vi "setup.vi"() -> (2 "Data":T1={"Report.lvclass"=refnum, "test"="", "last State"=enum."Initialize", "test ID"=0, "parameter"=[], "EMTestCWS500N.lvclass"=refnum, "CEG4500.lvclass"=refnum, "Tektronix RSA5106A.lvclass"=refnum, "erfolgreich"=FALSE, "log"="", "Kommentar"="", "Device Enum"=enum."emTestCWS500N", "Test Enum"=enum."HF-Felder", "debug"=FALSE}, 3 "reference":refnum<vi>)   [LabVIEW 2013]
uses:
  Main/controls/Data.ctl
  classes/Datastructure/Report/Report.lvclass
  classes/Devices/emTestCWS500N/EMTestCWS500N.lvclass
  classes/Devices/CEG4500/CEG4500.lvclass
  classes/Devices/Tektronix RSA5106A/Tektronix RSA5106A.lvclass
  Main/controls/State.ctl
  classes/Devices/DeviceInterface/Devices.ctl
  classes/Tests/TestInterface/Tests.ctl
  classes/Datastructure/Norm/Norm.lvclass
  classes/Datastructure/Test/Test.lvclass
  classes/Datastructure/Image/img.lvclass
  classes/Datastructure/Setup/Setup.lvclass
  classes/Datastructure/Device/Device.lvclass
panel:
  in  "gelesen von Datenstruktur":string(tree)
  out "Fehler (Ausgang)":errorcluster
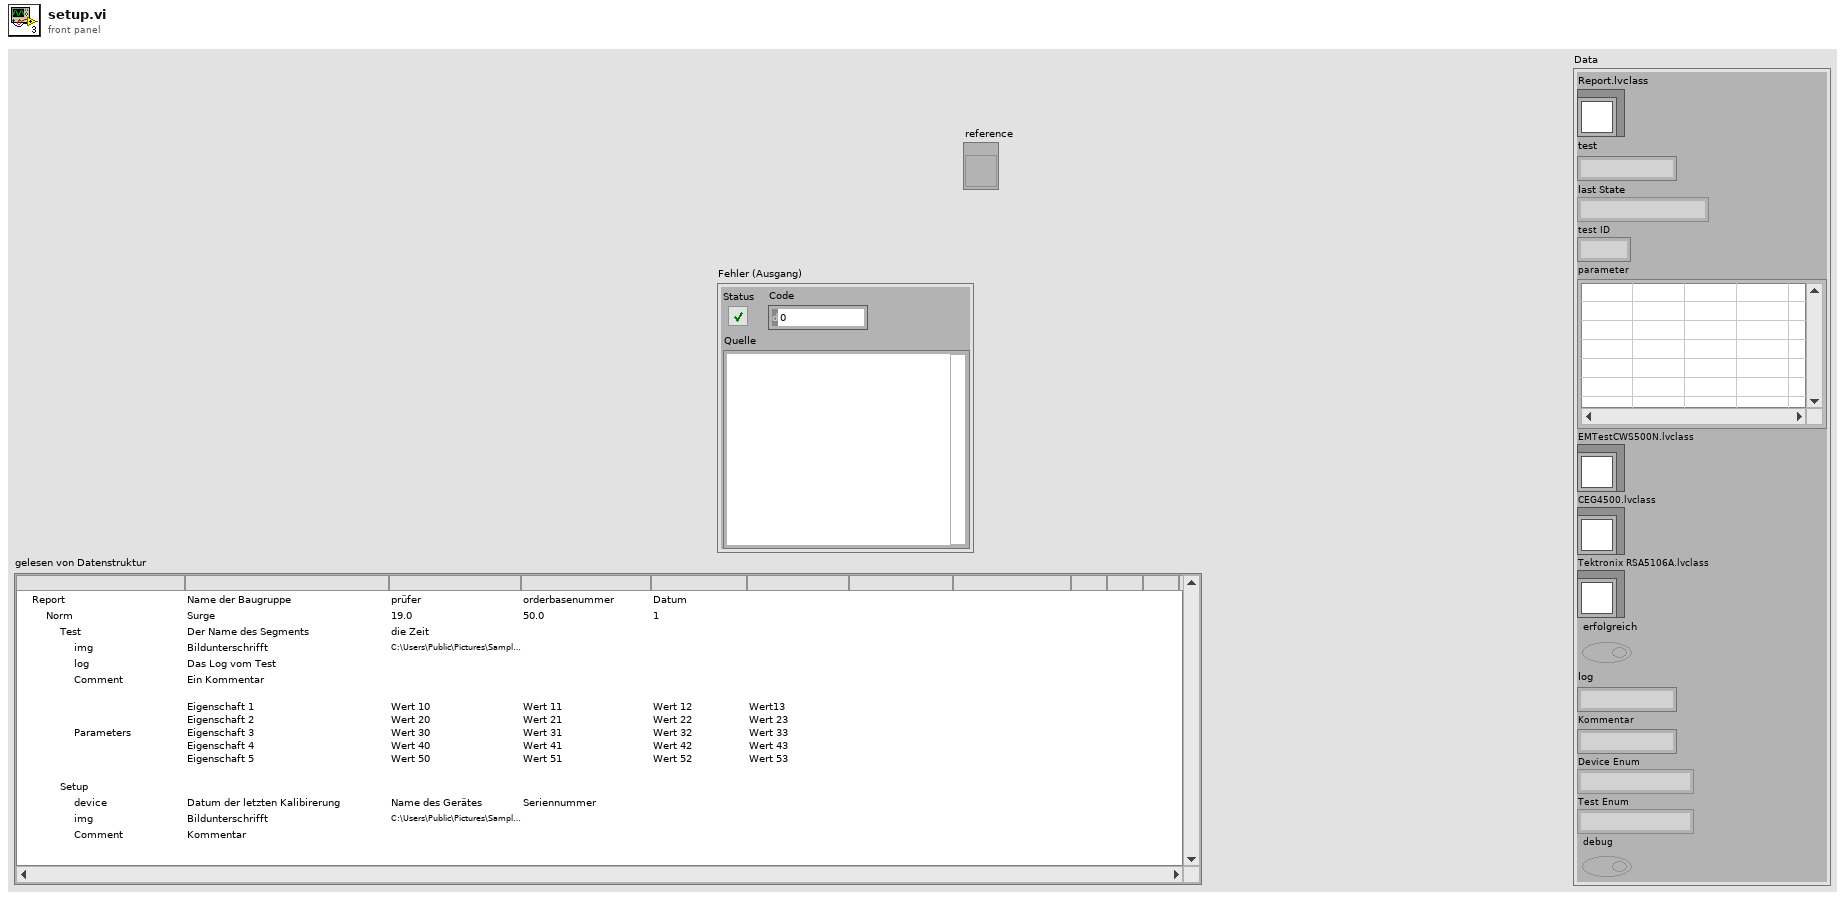
[diagram p1: front panel]
types:
  T1 = typedef "Data.ctl" = cluster{"Report.lvclass":refnum<class "Report.lvclass">, "test":string, "last State":T2, "test ID":i32, "parameter":string[][], "EMTestCWS500N.lvclass":refnum<class "EMTestCWS500N.lvclass">, "CEG4500.lvclass":refnum<class "CEG4500.lvclass">, "Tektronix RSA5106A.lvclass":refnum<class "Tektronix RSA5106A.lvclass">, "erfolgreich":bool, "log":string, "Kommentar":string, "Device Enum":T3, "Test Enum":T4, "debug":bool}
  T2 = typedef "State.ctl" = enum16{"create Pdf", "load Report", "save Report", "do Test", "CDN Kalibrierung", "enter Report Parameters", "new Test", "Protokoll", "read Tree", "update Tree", "Fehler", "Initialize", "Wait for Event", "Exit"}
  T3 = typedef "Devices.ctl" = enum16{"unbekannt", "Tektronix RSA5106A", "emTestCWS500N", "CEG-4500"}
  T4 = typedef "Tests.ctl" = enum16{"unbekannt", "Störaussendung", "Burst", "ESD", "Surge", "Spannungseinbruch", "HF-Felder"}
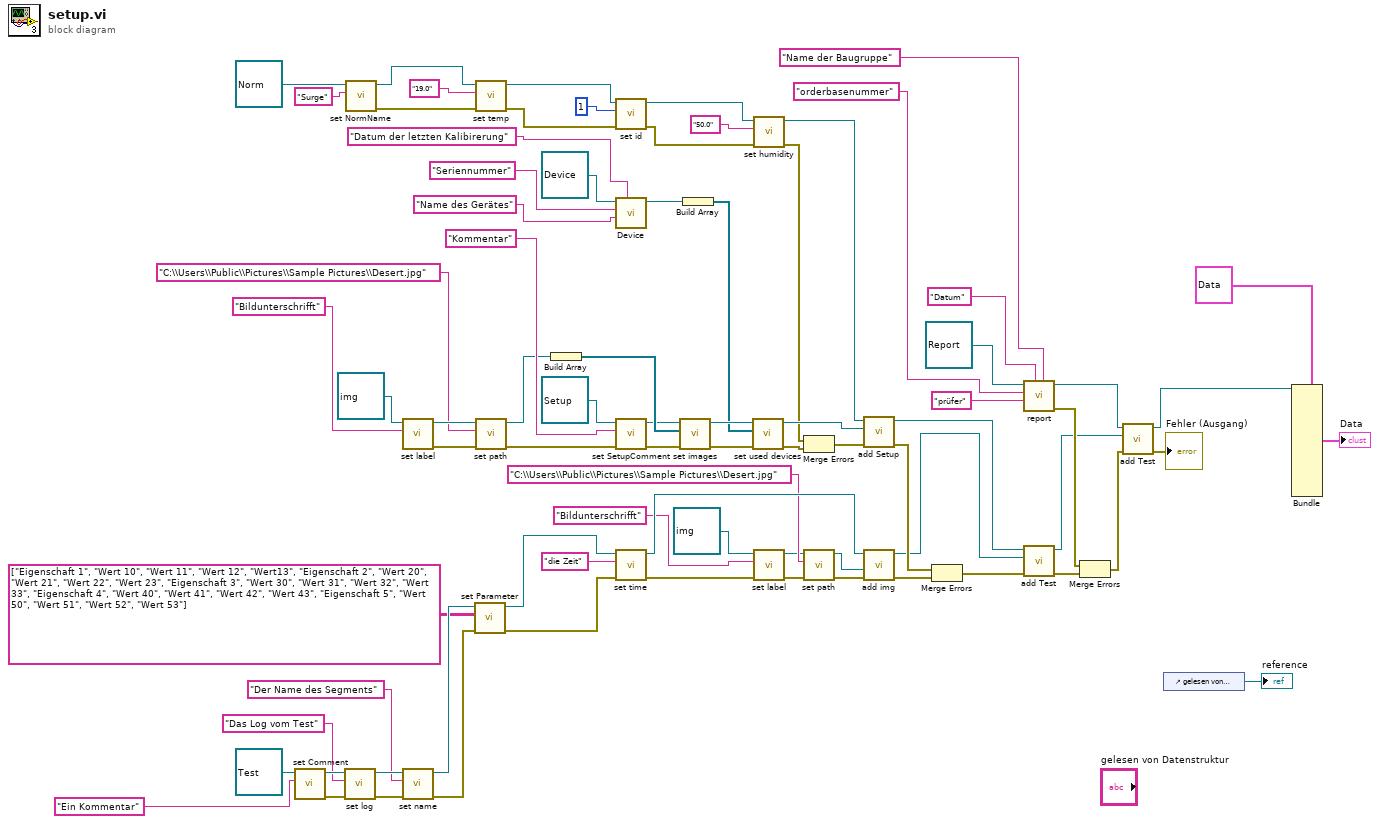
[diagram p0: block diagram]
diagram:
  n1 = call-dynamic "set Comment.vi"("Comment"="Ein Kommentar", "Segment (Eingang)"=refnum<class "Test.lvclass"> refnum ("Segment.lvclass")) -> ("error out"=w57:errorcluster, "Segment (Ausgang)"=w64:refnum<class "Test.lvclass">)  [unwired: 8 in]
  n2 = call-dynamic "set log.vi"("error in (no error)"=w57, "log"="Das Log vom Test", "Segment (Eingang)"=w64) -> ("error out"=w58:errorcluster, "Segment (Ausgang)"=w63:refnum<class "Test.lvclass">)  [unwired: 7 in]
  n3 = call-dynamic "set NormName.vi"("name"="Surge", "Test (Eingang)"=refnum<class "Norm.lvclass"> refnum ("Test.lvclass")) -> ("error out"=w8:errorcluster, "Test (Ausgang)"=w9:refnum<class "Norm.lvclass">)  [unwired: 8 in]
  n4 = call-dynamic "set label.vi"("label"="Bildunterschrifft", "img (Eingang)"=refnum<class "img.lvclass"> refnum ("img.lvclass")) -> ("error out"=w42:errorcluster, "img (Ausgang)"=w41:refnum<class "img.lvclass">)  [unwired: 8 in]
  n5 = call-dynamic "set name.vi"("error in (no error)"=w58, "name"="Der Name des Segments", "Segment (Eingang)"=w63) -> ("error out"=w59:errorcluster, "Segment (Ausgang)"=w62:refnum<class "Test.lvclass">)  [unwired: 7 in]
  n6 = call-dynamic "set Parameter.vi"("error in (no error)"=w59, "Parameter"=string[][] [["Eigenschaft 1", "Wert 10", "Wert 11", "Wert 12", "Wert13"], ["Eigenschaft 2", "Wert 20", "Wert 21", "Wert 22", "Wert 23"], ["Eigenschaft 3", "Wert 30", "Wert 31", "Wert 32", "Wert 33"], ["Eigenschaft 4", "Wert 40", "Wert 41", "Wert 42", "Wert 43"], ["Eigenschaft 5", "Wert 50", "Wert 51", "Wert 52", "Wert 53"]], "Segment (Eingang)"=w62) -> ("error out"=w60:errorcluster, "Segment (Ausgang)"=w61:refnum<class "Test.lvclass">)  [unwired: 7 in]
  n7 = call-dynamic "set temp.vi"("error in (no error)"=w8, "temp"="19.0", "Test (Eingang)"=w9) -> ("error out"=w71:errorcluster, "Test (Ausgang)"=w73:refnum<class "Norm.lvclass">)  [unwired: 7 in]
  n8 = call-dynamic "set path.vi"("error in (no error)"=w42, "path"="C:\\Users\\Public\\Pictures\\Sample Pictures\\Desert.jpg", "img (Eingang)"=w41) -> ("error out"=w17:errorcluster, "img (Ausgang)"=w34:refnum<class "img.lvclass">)  [unwired: 7 in]
  n9 = Build Array(w34) -> (w33:refnum<class "img.lvclass">[])
  n10 = call-dynamic "set id.vi"("error in (no error)"=w71, "id"=1, "Test (Eingang)"=w73) -> ("error out"=w70:errorcluster, "Test (Ausgang)"=w72:refnum<class "Norm.lvclass">)  [unwired: 7 in]
  n11 = call-dynamic "Device.vi"("last calibration"="Datum der letzten Kalibirerung", "Name"="Name des Gerätes", "serial"="Seriennummer", "Device Eingang"=refnum<class "Device.lvclass"> refnum ("Device.lvclass")) -> ("Device Ausgang"=w25:refnum<class "Device.lvclass">)  [unwired: 6 in, 1 out]
  n12 = call-dynamic "set SetupComment.vi"("error in (no error)"=w17, "Comment"="Kommentar", "Setup (Eingang)"=refnum<class "Setup.lvclass"> refnum ("Setup.lvclass")) -> ("error out"=w35:errorcluster, "Setup (Ausgang)"=w32:refnum<class "Setup.lvclass">)  [unwired: 7 in]
  n13 = call-dynamic "set time.vi"("error in (no error)"=w60, "time"="die Zeit", "Segment (Eingang)"=w61) -> ("error out"=w43:errorcluster, "Segment (Ausgang)"=w51:refnum<class "Test.lvclass">)  [unwired: 7 in]
  n14 = call-dynamic "set images.vi"("error in (no error)"=w35, "images"=w33, "Setup (Eingang)"=w32) -> ("error out"=w31:errorcluster, "Setup (Ausgang)"=w30:refnum<class "Setup.lvclass">)  [unwired: 7 in]
  n15 = Build Array(w25) -> (w24:refnum<class "Device.lvclass">[])
  n16 = call-dynamic "set used devices.vi"("error in (no error)"=w31, "used devices"=w24, "Setup (Eingang)"=w30) -> ("error out"=w21:errorcluster, "Setup (Ausgang)"=w23:refnum<class "Setup.lvclass">)  [unwired: 7 in]
  n17 = call-dynamic "set humidity.vi"("error in (no error)"=w70, "humidity"="50.0", "Test (Eingang)"=w72) -> ("error out"=w22:errorcluster, "Test (Ausgang)"=w66:refnum<class "Norm.lvclass">)  [unwired: 7 in]
  n18 = call-dynamic "set label.vi"("error in (no error)"=w43, "label"="Bildunterschrifft", "img (Eingang)"=refnum<class "img.lvclass"> refnum ("img.lvclass")) -> ("error out"=w44:errorcluster, "img (Ausgang)"=w47:refnum<class "img.lvclass">)  [unwired: 7 in]
  n19 = Merge Errors(w22, w21) -> (w20:errorcluster)
  n20 = call-dynamic "set path.vi"("error in (no error)"=w44, "path"="C:\\Users\\Public\\Pictures\\Sample Pictures\\Desert.jpg", "img (Eingang)"=w47) -> ("error out"=w45:errorcluster, "img (Ausgang)"=w46:refnum<class "img.lvclass">)  [unwired: 7 in]
  n21 = call-dynamic "add Setup.vi"("error in (no error)"=w20, "Setup"=w23, "Test Eingang"=w66) -> ("error out"=w19:errorcluster, "Test Ausgang"=w14:refnum<class "Norm.lvclass">)  [unwired: 7 in]
  n22 = call-dynamic "add img.vi"("error in (no error)"=w45, "img.lvclass"=w46, "Segment (Eingang)"=w51) -> ("error out"=w18:errorcluster, "Segment (Ausgang)"=w13:refnum<class "Test.lvclass">)  [unwired: 6 in]
  n23 = Merge Errors(w19, w18) -> (w12:errorcluster)
  n24 = call-dynamic "report.vi"("Rname"="Name der Baugruppe", "date"="Datum", "pruefer"="prüfer", "obnr"="orderbasenummer", "Report in"=refnum<class "Report.lvclass"> refnum ("Report.lvclass")) -> ("error out"=w16:errorcluster, "Report out"=w78:refnum<class "Report.lvclass">)  [unwired: 5 in]
  n25 = call-dynamic "add Test.vi"("error in (no error)"=w12, "Segment.lvclass"=w13, "Test Eingang"=w14) -> ("error out"=w11:errorcluster, "Test Ausgang"=w10:refnum<class "Norm.lvclass">)  [unwired: 7 in]
  n26 = Merge Errors(w16, w11) -> (w15:errorcluster)
  n27 = call-dynamic "add Test.vi"("error in (no error)"=w15, "Test.lvclass"=w10, "Report (Eingang)"=w78) -> ("error out"=→"Fehler (Ausgang)":errorcluster, "Report (Ausgang)"=w3:refnum<class "Report.lvclass">)  [unwired: 7 in]
  n28 = control-ref of="gelesen von Datenstruktur"() -> (→"reference":refnum<vi>)
  n29 = Bundle(cluster=T1 {"Report.lvclass"=refnum, "test"="", "last State"=enum."Initialize", "test ID"=0, "parameter"=[], "EMTestCWS500N.lvclass"=refnum, "CEG4500.lvclass"=refnum, "Tektronix RSA5106A.lvclass"=refnum, "erfolgreich"=FALSE, "log"="", "Kommentar"="", "Device Enum"=enum."emTestCWS500N", "Test Enum"=enum."HF-Felder", "debug"=FALSE} ("Daten"), "Report.lvclass"=w3) -> (→"Data":T1)  [unwired: 13 in]
